vi "find_vertex_min_max.vi"(10 "Total Range Min/Max":T1, 11 "Vertex Array":cluster{"X":sgl, "Y":sgl, "Z":sgl}[](array[cluster])) -> (2 "Total Range Out":T1, 3 "This Range Min/Max Out":T1)   [LabVIEW 2020]
uses:
  <vilib>/Native 3D Graph/typedefs/range_cluster.ctl
  <vilib>/Native 3D Graph/typedefs/min_max.ctl
  <vilib>/Native 3D Graph/xcontrol/3DPC_SurfacePlot.xctl
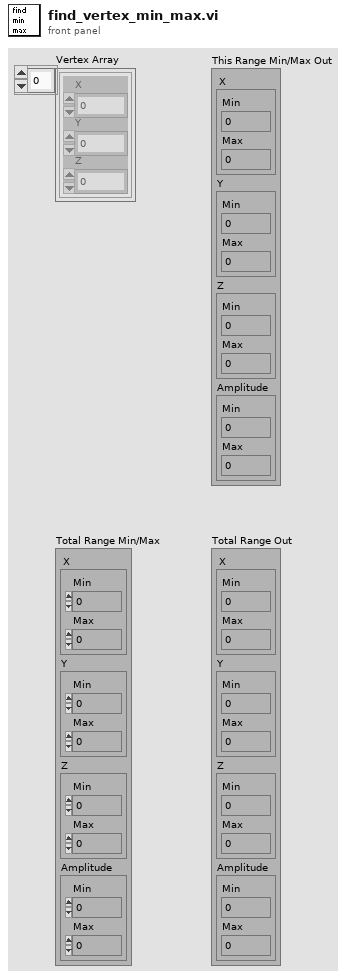
[diagram p1: front panel]
types:
  T1 = typedef "3DPC_SurfacePlot.xctl/range_cluster.ctl" = cluster{"X":T2, "Y":T2, "Z":T2, "Amplitude":T2}
  T2 = typedef "3DPC_SurfacePlot.xctl/min_max.ctl" = cluster{"Min":sgl, "Max":sgl}
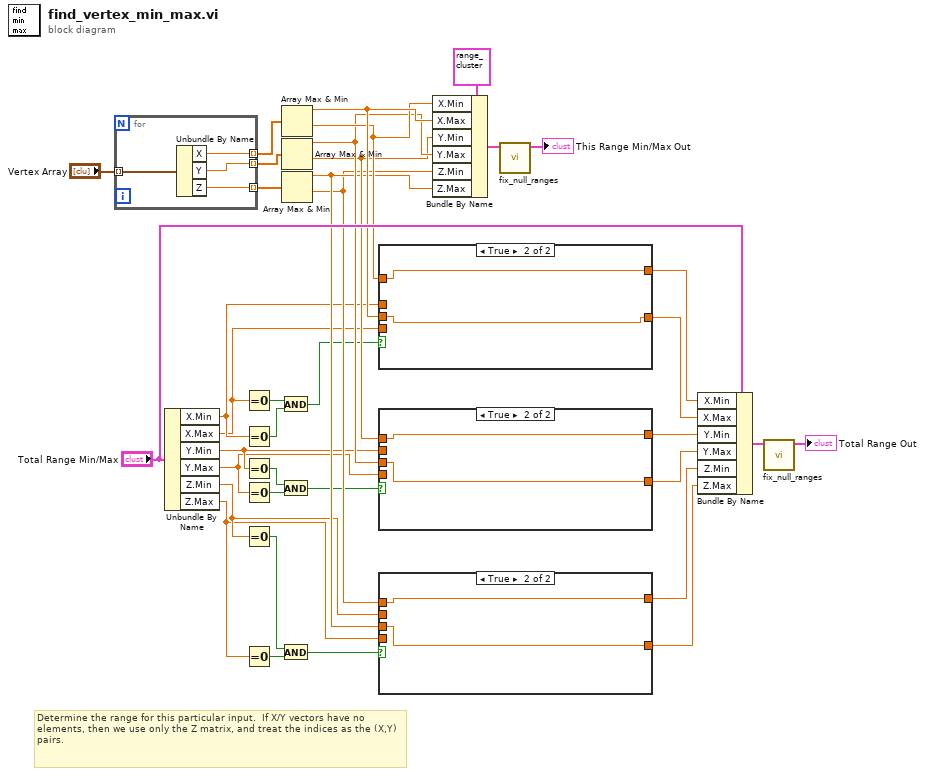
[diagram p0: block diagram]
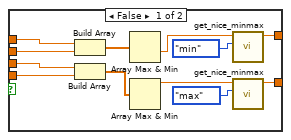
[diagram p2: hidden frame]
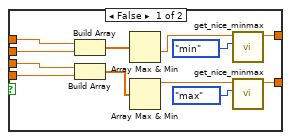
[diagram p3: hidden frame]
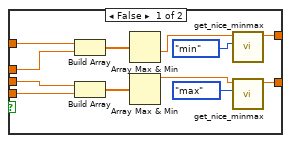
[diagram p4: hidden frame]
diagram:
  # "Determine the range for this particular input.  If X/Y vectors have no elements, then we use only the Z matrix, and treat the indices as the (X,Y) pairs."
  n1 = for {
    tunnel: "Vertex Array" -> [w41] mode=indexing
    tunnel: [w40] -> w36 mode=indexing
    tunnel: [w39] -> w35 mode=indexing
    tunnel: [w38] -> w34 mode=indexing
    n2 = Unbundle By Name(w41) -> ("X"=w40:sgl, "Y"=w39:sgl, "Z"=w38:sgl)
  }
  n3 = Unbundle By Name("Total Range Min/Max") -> ("X.Min"=w15:sgl, "X.Max"=w14:sgl, "Y.Min"=w7:sgl, "Y.Max"=w6:sgl, "Z.Min"=w4:sgl, "Z.Max"=w3:sgl)
  n4 = Equal To 0?(x=w14) -> (x = 0?=w12:bool)
  n5 = Equal To 0?(x=w15) -> (x = 0?=w13:bool)
  n6 = Equal To 0?(x=w7) -> (x = 0?=w10:bool)
  n7 = Equal To 0?(x=w6) -> (x = 0?=w9:bool)
  n8 = Equal To 0?(x=w4) -> (x = 0?=w5:bool)
  n9 = Equal To 0?(x=w3) -> (x = 0?=w2:bool)
  n10 = And(x=w12, y=w13) -> (x .and. y?=w11:bool)
  n11 = And(x=w10, y=w9) -> (x .and. y?=w8:bool)
  n12 = And(x=w5, y=w2) -> (x .and. y?=w1:bool)
  n13 = Array Max & Min(array=w36) -> (max value=w25:sgl, min value=w24:sgl)  [unwired: 2 out]
  n14 = Array Max & Min(array=w35) -> (max value=w23:sgl, min value=w22:sgl)  [unwired: 2 out]
  n15 = Array Max & Min(array=w34) -> (max value=w21:sgl, min value=w20:sgl)  [unwired: 2 out]
  n16 = case shown="True" w11 {
    tunnel: w15 -> [w53 _]
    tunnel: w14 -> [w50 _]
    tunnel: [w48 w55] -> w31
    tunnel: [w46 w54] -> w30
    tunnel: w25 -> [w43 w54]
    tunnel: w24 -> [w42 w55]
    frame False {
      n17 = Build Array(w42, w53) -> (w52:sgl[])
      n18 = Build Array(w43, w50) -> (w51:sgl[])
      n19 = Array Max & Min(array=w52) -> (min value=w49:sgl)  [unwired: 3 out]
      n20 = Array Max & Min(array=w51) -> (max value=w47:sgl)  [unwired: 3 out]
      n21 = call <vilib>:"get_nice_minmax.vi"("Enum"=enum16{"min", "max"}."min", "input"=w49) -> ("output"=w48:sgl)  [unwired: 9 out]
      n22 = call <vilib>:"get_nice_minmax.vi"("Enum"=enum16{"min", "max"}."max", "input"=w47) -> ("output"=w46:sgl)  [unwired: 9 out]
    }
    frame True {
    }
  }
  n23 = case shown="True" w8 {
    tunnel: w7 -> [w65 _]
    tunnel: w6 -> [w64 _]
    tunnel: [w62 w69] -> w29
    tunnel: [w61 w68] -> w28
    tunnel: w23 -> [w59 w68]
    tunnel: w22 -> [w58 w69]
    frame False {
      n24 = Build Array(w58, w65) -> (w67:sgl[])
      n25 = Build Array(w59, w64) -> (w66:sgl[])
      n26 = Array Max & Min(array=w67) -> (min value=w63:sgl)  [unwired: 3 out]
      n27 = Array Max & Min(array=w66) -> (max value=w60:sgl)  [unwired: 3 out]
      n28 = call <vilib>:"get_nice_minmax.vi"("Enum"=enum16{"min", "max"}."min", "input"=w63) -> ("output"=w62:sgl)  [unwired: 9 out]
      n29 = call <vilib>:"get_nice_minmax.vi"("Enum"=enum16{"min", "max"}."max", "input"=w60) -> ("output"=w61:sgl)  [unwired: 9 out]
    }
    frame True {
    }
  }
  n30 = case shown="True" w1 {
    tunnel: w4 -> [w79 _]
    tunnel: w3 -> [w78 _]
    tunnel: [w76 w83] -> w27
    tunnel: [w74 w82] -> w26
    tunnel: w21 -> [w73 w82]
    tunnel: w20 -> [w72 w83]
    frame False {
      n31 = Build Array(w72, w79) -> (w81:sgl[])
      n32 = Build Array(w73, w78) -> (w80:sgl[])
      n33 = Array Max & Min(array=w81) -> (min value=w77:sgl)  [unwired: 3 out]
      n34 = Array Max & Min(array=w80) -> (max value=w75:sgl)  [unwired: 3 out]
      n35 = call <vilib>:"get_nice_minmax.vi"("Enum"=enum16{"min", "max"}."min", "input"=w77) -> ("output"=w76:sgl)  [unwired: 9 out]
      n36 = call <vilib>:"get_nice_minmax.vi"("Enum"=enum16{"min", "max"}."max", "input"=w75) -> ("output"=w74:sgl)  [unwired: 9 out]
    }
    frame True {
    }
  }
  n37 = Bundle By Name(cluster=T1 {"X"={"Min"=0.0, "Max"=0.0}, "Y"={"Min"=0.0, "Max"=0.0}, "Z"={"Min"=0.0, "Max"=0.0}, "Amplitude"={"Min"=0.0, "Max"=0.0}} ("This Range Min/Max Out"), "X.Min"=w24, "X.Max"=w25, "Y.Min"=w22, "Y.Max"=w23, "Z.Min"=w20, "Z.Max"=w21) -> (w19:T1)
  n38 = call <vilib>:"fix_null_ranges.vi"("input cluster"=w19) -> ("output cluster"=→"This Range Min/Max Out":T1)  [unwired: 10 out]
  n39 = Bundle By Name(cluster="Total Range Min/Max", "X.Min"=w31, "X.Max"=w30, "Y.Min"=w29, "Y.Max"=w28, "Z.Min"=w27, "Z.Max"=w26) -> (w17:T1)
  n40 = call <vilib>:"fix_null_ranges.vi"("input cluster"=w17) -> ("output cluster"=→"Total Range Out":T1)  [unwired: 10 out]
